vi "Lab_Dummy.vi"(6 "Unused Input 5":dbl, 8 "Unused Input 4":dbl, 9 "Unused Input 3":dbl, 10 "Unused Input 2":dbl, 11 "Unused Input 1":string) -> (1 "Time":dbl[](array[numeric]), 2 "Vout":dbl[](array[numeric]), 3 "Vin":dbl[](array[numeric]))   [LabVIEW 2013]
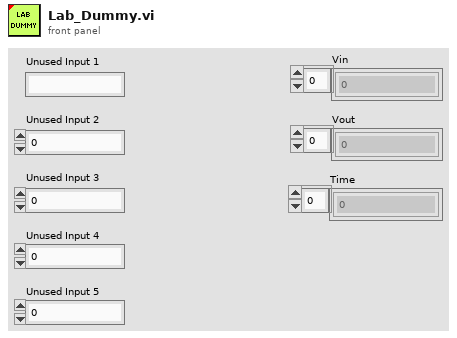
[diagram p1: front panel]
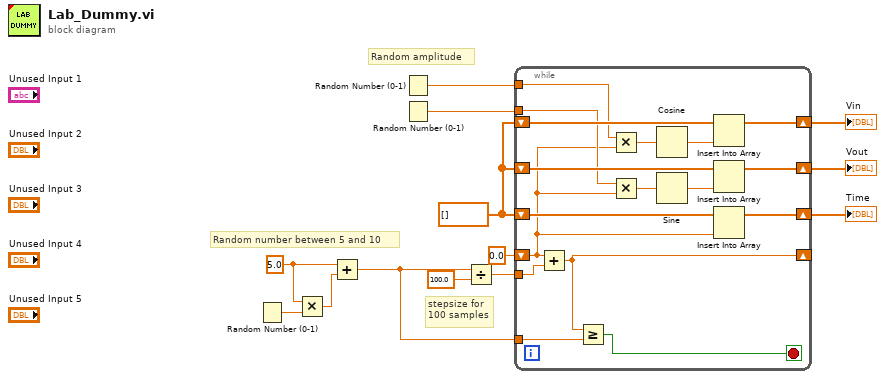
[diagram p0: block diagram]
diagram:
  w13 = 5.0 ("x")
  w6 = dbl[] []
  # "Random amplitude"
  # "stepsize for\n100 samples"
  # "Random number between 5 and 10"
  n1 = Random Number (0-1)() -> (number: 0 to 1=w12:dbl)
  n2 = Multiply(x=w13, y=w12) -> (x*y=w11:dbl)
  n3 = Add(x=w13, y=w11) -> (x+y=w7:dbl)
  n4 = Random Number (0-1)() -> (number: 0 to 1=w1:dbl)
  n5 = Random Number (0-1)() -> (number: 0 to 1=w2:dbl)
  n6 = Divide(x=w7, y=100.0) -> (x/y=w9:dbl)
  n7 = while {
    tunnel: w9 -> [w30]
    shift-right: [w29] -> _
    shift-left: 0.0 -> [w14]
    tunnel: w7 -> [w28]
    shift-right: [w26] -> w3
    shift-left: w6 -> [w27]
    shift-right: [w23] -> w4
    shift-left: w6 -> [w24]
    shift-right: [w19] -> w5
    shift-left: w6 -> [w20]
    tunnel: w2 -> [w16]
    tunnel: w1 -> [w15]
    stop <- w25 stop-if-true
    n8 = Add(x=w14, y=w30) -> (x+y=w29:dbl)
    n9 = Greater Or Equal?(x=w29, y=w28) -> (x >= y?=w25:bool)
    n10 = Multiply(x=w15, y=w14) -> (x*y=w18:dbl)
    n11 = Multiply(x=w16, y=w14) -> (x*y=w17:dbl)
    n12 = Cosine(x=w18) -> (cos(x)=w21:dbl)
    n13 = Sine(x=w17) -> (sin(x)=w22:dbl)
    n14 = Insert Into Array(array=w20, new element=w21) -> (w19:dbl[])  [unwired: 1 in]
    n15 = Insert Into Array(array=w24, new element=w22) -> (w23:dbl[])  [unwired: 1 in]
    n16 = Insert Into Array(array=w27, new element=w14) -> (w26:dbl[])  [unwired: 1 in]
  }
  "Time" <- w3
  "Vin" <- w5
  "Vout" <- w4
